vi "Keep Pose.vi"(6 "Encoder Right":dbl, 7 "Encoder Left":dbl, 8 "Right Axis":dbl, 9 "Left Axis":dbl, 10 "Angle":dbl, 11 "Keep Pose":bool) -> (0 "Right":dbl, 1 "Left":dbl)   [LabVIEW 2015]
uses:
  <vilib>/addons/control/pid/pid.llb/PID (DBL).vi
  <vilib>/addons/control/pid/NI_PID_pid.lvlib
panel:
  in  "PID Drive":T1={"proportional gain (Kc)"=-0.2, "integral time (Ti, min)"=0.0, "derivative time (Td, min)"=0.0} {"derivative time (Td, min)" format="%.3f"; "integral time (Ti, min)" format="%.3f"; "proportional gain (Kc)" format="%.3f"}
  in  "PID Angle":T1={"proportional gain (Kc)"=-0.1, "integral time (Ti, min)"=0.0, "derivative time (Td, min)"=0.0}
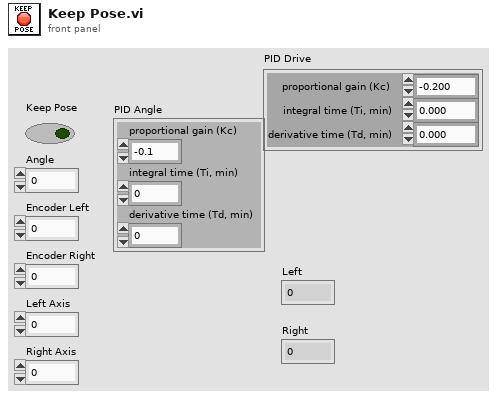
[diagram p1: front panel]
types:
  T1 = cluster{"proportional gain (Kc)":dbl, "integral time (Ti, min)":dbl, "derivative time (Td, min)":dbl}
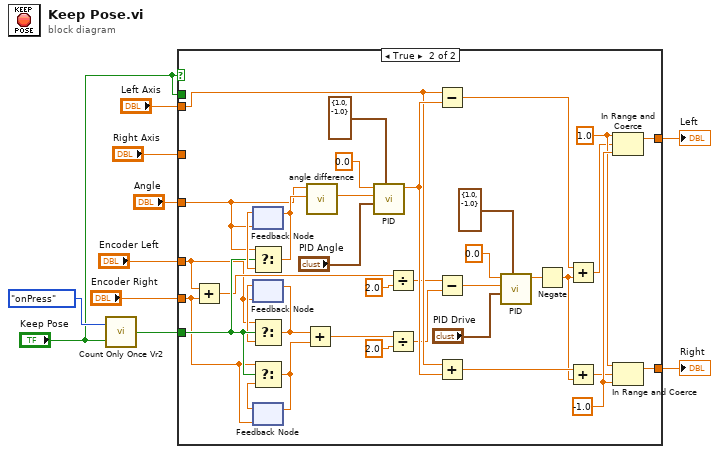
[diagram p0: block diagram]
diagram:
  n1 = call "Count Only Once Vr2.vi"("InValue"="Keep Pose", "Action"=enum16{"onPress", "onRelease", "Both"}."onPress") -> ("Result"=w7:bool)
  n2 = case shown="True" "Keep Pose" {
    tunnel: [w12 w42] -> w10
    tunnel: [w11 w41] -> w9
    tunnel: "Keep Pose" -> [_ _]
    tunnel: "Left Axis" -> [w12 w40]
    tunnel: "Right Axis" -> [w11 _]
    tunnel: w7 -> [_ w35]
    tunnel: "Angle" -> [_ w36]
    tunnel: "Encoder Right" -> [_ w14]
    tunnel: "Encoder Left" -> [_ w26]
    frame False {
    }
    frame True {
      w45 = -1.0 ("lower limit")
      w44 = 1.0 ("upper limit")
      n3 = Add(x=w26, y=w14) -> (x+y=w28:dbl)
      n4 = feedback #1(w36) -> (w48:dbl)
      n5 = Select(t=w36, s=w35, f=w48) -> (s? t:f=w39:dbl)
      n6 = feedback-in #1(w39) -> ()
      n7 = feedback #2(w26) -> (w34:dbl)
      n8 = Select(t=w26, s=w35, f=w34) -> (s? t:f=w31:dbl)
      n9 = feedback-in #2(w31) -> ()
      n10 = feedback #3(w14) -> (w33:dbl)
      n11 = Select(t=w14, s=w35, f=w33) -> (s? t:f=w32:dbl)
      n12 = feedback-in #3(w32) -> ()
      n13 = Add(x=w31, y=w32) -> (x+y=w30:dbl)
      n14 = call "angle difference.vi"("angle2"=w39, "angle1"=w36) -> ("angle diff"=w46:dbl)  [unwired: 9 in]
      n15 = call-poly <vilib>:"PID.vi"("output range"=cluster{"output high":dbl, "output low":dbl} {"output high"=1.0, "output low"=-1.0}, "PID gains"="PID Angle", "process variable"=w46, "setpoint"=0.0) -> ("output"=w43:dbl)  [unwired: 6 in, 1 out]
      n16 = Divide(x=w28, y=2.0) -> (x/y=w25:dbl)
      n17 = Divide(x=w30, y=2.0) -> (x/y=w24:dbl)
      n18 = Subtract(x=w40, y=w43) -> (x-y=w23:dbl)
      n19 = Subtract(x=w25, y=w24) -> (x-y=w16:dbl)
      n20 = Add(x=w40, y=w43) -> (x+y=w21:dbl)
      n21 = call-poly <vilib>:"PID.vi"("output range"=cluster{"output high":dbl, "output low":dbl} {"output high"=1.0, "output low"=-1.0}, "PID gains"="PID Drive", "process variable"=w16, "setpoint"=0.0) -> ("output"=w19:dbl)  [unwired: 6 in, 1 out]
      n22 = Negate(x=w19) -> (-x=w13:dbl)
      n23 = Add(x=w23, y=w13) -> (x+y=w22:dbl)
      n24 = Add(x=w21, y=w13) -> (x+y=w20:dbl)
      n25 = In Range and Coerce(upper limit=w44, x=w22, lower limit=w45) -> (coerced(x)=w42:dbl)  [unwired: 1 out]
      n26 = In Range and Coerce(upper limit=w44, x=w20, lower limit=w45) -> (coerced(x)=w41:dbl)  [unwired: 1 out]
    }
  }
  "Left" <- w10
  "Right" <- w9
